vi "get_string_value_array.vi"(3 "error in (no error)":errorcluster, 4 "field name":string, 5 "metadata JSON string":string) -> (0 "error out":errorcluster, 2 "string array":string[](array[string]))   [LabVIEW 2013]
uses:
  <vilib>/LVH/i3 JSON/JSON Parsing/Get Object Parameter Files/Get Object Parameter - Array.vi
  <vilib>/LVH/i3 JSON/JSON Parsing/Get Array Value at Index Files/Get Array Value at Index - String.vi
  i3 JSON/i3-json.lvlib
panel:
  out "JSON Tree":variant
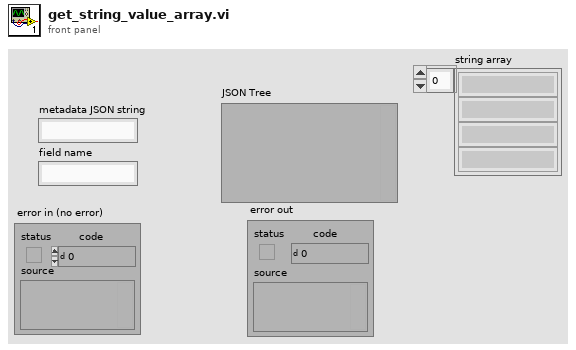
[diagram p1: front panel]
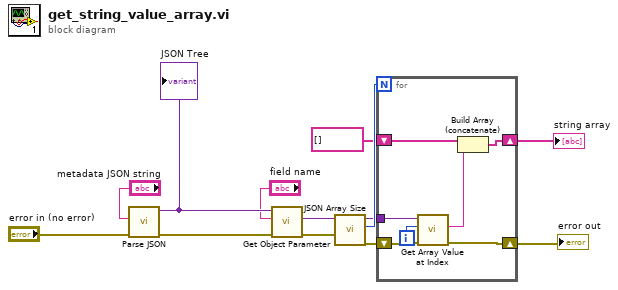
[diagram p0: block diagram]
diagram:
  n1 = call <vilib>:"Parse JSON.vi"("error in (no error)"="error in (no error)", "JSON String"="metadata JSON string") -> ("error out"=w11:errorcluster, "JSON Tree"=w12:variant)  [unwired: 6 in, 2 out]
  "JSON Tree" <- w12
  n2 = call-poly <vilib>:"Get Object Parameter.vi"("error in (no error)"=w11, "Parameter Name"="field name", "JSON Tree In (JSON Object)"=w12) -> ("error out"=w6:errorcluster, "JSON Array"=w8:variant)  [unwired: 5 in, 2 out]
  n3 = call <vilib>:"JSON Array Size.vi"("error in (no error)"=w6, "JSON Tree In (JSON Array)"=w8) -> ("error out"=w4:errorcluster, "Array Size"=w7:i32, "JSON Tree Passthrough (JSON Array)"=w5:variant)  [unwired: 7 in]
  n4 = for {
    N: w7 -> [_]
    tunnel: w5 -> [w20]
    shift-right: [w14] -> w3
    shift-left: w4 -> [w18]
    shift-right: [w15] -> w1
    shift-left: string[] [] ("string array 2") -> [w16]
    i -> [w19]
    n5 = call-poly <vilib>:"Get Array Value at Index.vi"("error in (no error)"=w18, "Index"=w19, "JSON Tree In (JSON Array)"=w20) -> ("error out"=w14:errorcluster, "String Value"=w17:string)  [unwired: 5 in, 2 out]
    n6 = Build Array (concatenate)(w16, w17) -> (w15:string[])
  }
  "string array" <- w1
  "error out" <- w3
